vi "Publish Group.vi"(8 "error in (no error)":errorcluster, 10 "Group":refnum<class "GroupAbstract.lvclass">, 11 "TelemetryAPI in":refnum<class "TelemetryAPI.lvclass">) -> (0 "error out":errorcluster, 3 "TelemetryAPI out":refnum<class "TelemetryAPI.lvclass">)   [LabVIEW 2020, in "Volatus.lvlib" / "TelemetryAPI.lvclass"]
uses:
  TelemetryAPI.lvclass
  TelemetryAPI.lvclass/TelemetryAPI.ctl
  lv-vecto/Vecto/RemoteDataService/RemoteDataService.lvclass
  lv-vecto/Vecto/GroupAbstract/GroupAbstract.lvclass
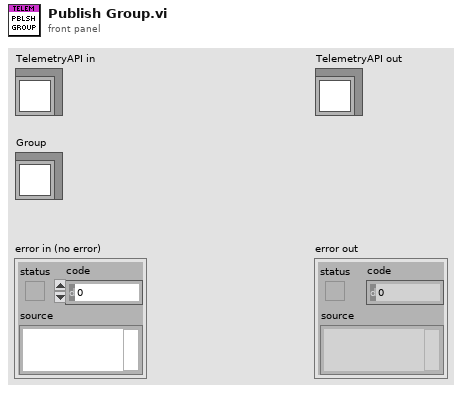
[diagram p1: front panel]
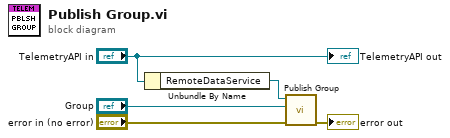
[diagram p0: block diagram]
diagram:
  n1 = Unbundle By Name("TelemetryAPI in") -> ("RemoteDataService"=w4:refnum<class "RemoteDataService.lvclass">)
  n2 = call "Publish Group.vi"("error in (no error)"="error in (no error)", "Group"="Group", "RemoteDataService in"=w4) -> ("error out"=→"error out":errorcluster)  [unwired: 7 in, 1 out]
  "TelemetryAPI out" <- "TelemetryAPI in"
